vi "Gap Between CNTs.vi"(10 "m-nm Gap":dbl, 11 "Gap Between CNTs":dbl) -> (3 "Numeric":dbl)   [LabVIEW 2020]
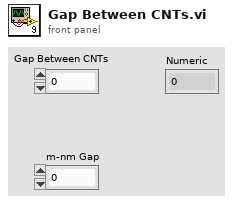
[diagram p1: front panel]
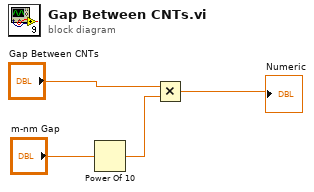
[diagram p0: block diagram]
diagram:
  n1 = Power Of 10(x="m-nm Gap") -> (10^x=w3:dbl)
  n2 = Multiply(x="Gap Between CNTs", y=w3) -> (x*y=→"Numeric":dbl)
